vi "Select_Value.vi"(2 "Numerisch":i32, 3 "System Monitor Variables":T1) -> (0 "Array":dbl[](array[numeric]), 1 "Value":dbl format="%#_13g")   [LabVIEW 2016]
uses:
  Global/Global Variables/System Monitor Cluster.ctl
panel:
  out "String":string
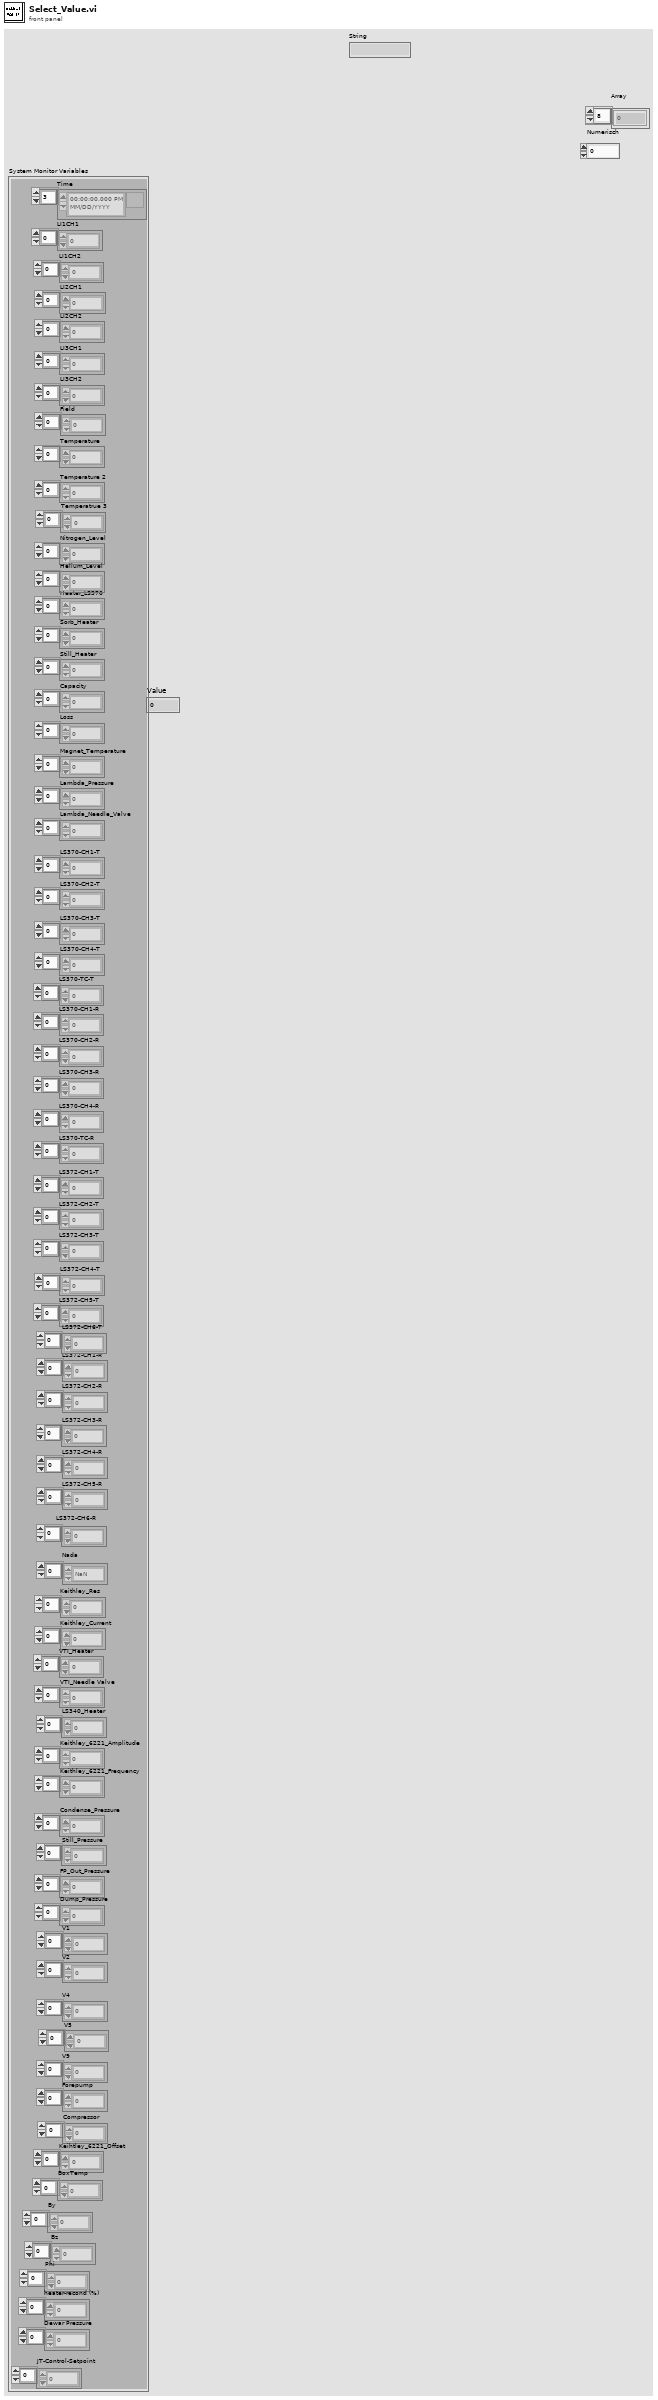
[diagram p1: front panel]
types:
  T1 = typedef "System Monitor Cluster.ctl" = cluster{"Time":timestamp[], "LI1CH1":dbl[], "LI1CH2":dbl[], "LI2CH1":dbl[], "LI2CH2":dbl[], "LI3CH1":dbl[], "LI3CH2":dbl[], "Field":dbl[], "Temperature":dbl[], "Temperature 2":dbl[], "Temperatrue 3":dbl[], "Nitrogen_Level":dbl[], "Helium_Level":dbl[], "Heater_LS370":dbl[], "Sorb_Heater":dbl[], "Still_Heater":dbl[], "Capacity":dbl[], "Loss":dbl[], "Magnet_Temperature":dbl[], "Lambda_Pressure":dbl[], "Lambda_Needle_Valve":dbl[], "LS370-CH1-T":dbl[], "LS370-CH2-T":dbl[], "LS370-CH3-T":dbl[], "LS370-CH4-T":dbl[], "LS370-TC-T":dbl[], "LS370-CH1-R":dbl[], "LS370-CH2-R":dbl[], "LS370-CH3-R":dbl[], "LS370-CH4-R":dbl[], "LS370-TC-R":dbl[], "LS372-CH1-T":dbl[], "LS372-CH2-T":dbl[], "LS372-CH3-T":dbl[], "LS372-CH4-T":dbl[], "LS372-CH5-T":dbl[], "LS372-CH6-T":dbl[], "LS372-CH1-R":dbl[], "LS372-CH2-R":dbl[], "LS372-CH3-R":dbl[], "LS372-CH4-R":dbl[], "LS372-CH5-R":dbl[], "LS372-CH6-R":dbl[], "Nada":dbl[], "Keithley_Res":dbl[], "Keithley_Current":dbl[], "VTI_Heater":dbl[], "VTI_Needle Valve":dbl[], "LS340_Heater":dbl[], "Keithley_6221_Amplitude":dbl[], "Keithley_6221_Frequency":dbl[], "Condense_Pressure":dbl[], "Still_Pressure":dbl[], "FP_Out_Pressure":dbl[], "Dump_Pressure":dbl[], "V1":dbl[], "V2":dbl[], "V4":dbl[], "V5":dbl[], "V9":dbl[], "Forepump":dbl[], "Compressor":dbl[], "Keihtley_6221_Offset":dbl[], "BoxTemp":dbl[], "By":dbl[], "Bz":dbl[], "Phi":dbl[], "heater-recond (%)":dbl[], "Dewar Pressure ":dbl[], "JT-Control-Setpoint":dbl[]}
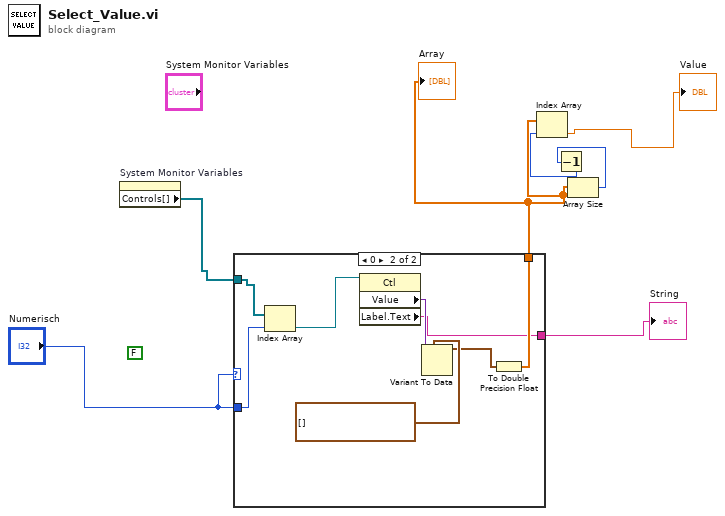
[diagram p0: block diagram]
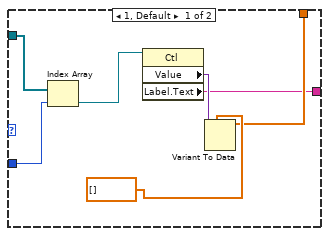
[diagram p2: hidden frame]
diagram:
  (unwired) FALSE
  n1 = property on="System Monitor Variables" class="Clust (strict)"() -> ("Controls[]"=w7:refnum<vi>[])  [unwired: 2 in, 2 out]
  n2 = case shown="0" "Numerisch" {
    tunnel: w7 -> [w12 w22]
    tunnel: "Numerisch" -> [w11 w20]
    tunnel: [w9 w17] -> w3
    tunnel: [w8 w16] -> w1
    frame 1, Default {
      n3 = Index Array(array=w12, index=w11) -> (element=w13:refnum<vi>)
      n4 = property class="Ctl"(reference=w13) -> ("Value"=w14:variant, "Label.Text"=w8:string)  [unwired: 1 in, 2 out]
      n5 = Variant To Data(type=dbl[] [] ("Array 3"), Variant=w14) -> (data=w9:dbl[])  [unwired: 1 in, 1 out]
    }
    frame 0 {
      n6 = Index Array(array=w22, index=w20) -> (element=w21:refnum<vi>)
      n7 = property class="Ctl"(reference=w21) -> ("Value"=w19:variant, "Label.Text"=w16:string)  [unwired: 1 in, 2 out]
      n8 = Variant To Data(type=timestamp[] [] ("Time"), Variant=w19) -> (data=w15:timestamp[])  [unwired: 1 in, 1 out]
      n9 = To Double Precision Float(number=w15) -> (double precision float=w17:dbl[])
    }
  }
  "Array" <- w3
  "String" <- w1
  n10 = Array Size(array=w3) -> (size(s)=w6:i32)
  n11 = Decrement(x=w6) -> (x-1=w5:i32)
  n12 = Index Array(array=w3, index=w5) -> (element=→"Value":dbl)
